vi "Laser Ethernet Rack_Init.vi"(0 "object in":refnum<class "Laser Ethernet Rack.lvclass">, 5 "error in (no error)":errorcluster) -> (14 "object out":refnum<class "Laser Ethernet Rack.lvclass">, 19 "error out":errorcluster)   [LabVIEW 2023, in "Laser Ethernet Rack.lvclass"]
uses:
  Laser Ethernet Rack.lvclass
  C:/Users/TimBerrier/Code/LabVIEW/Source/APIs/IPG/ipg_tcp/Laser_Ethernet_class/Laser_Ethernet.lvclass
  Laser Ethernet Rack.lvclass/Laser Ethernet Rack.ctl
  Laser_Ethernet_class/Laser_Ethernet.lvclass
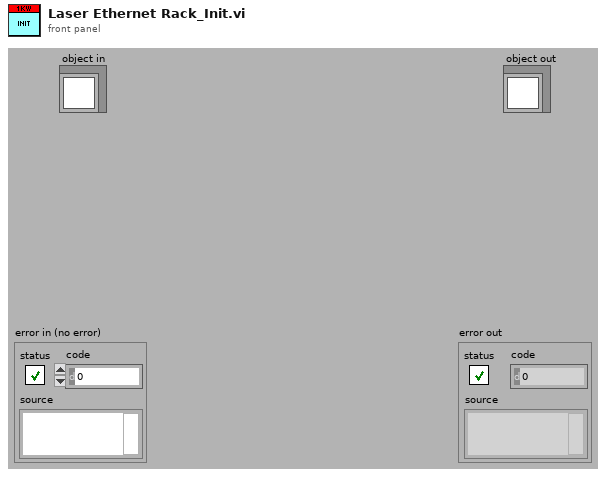
[diagram p1: front panel]
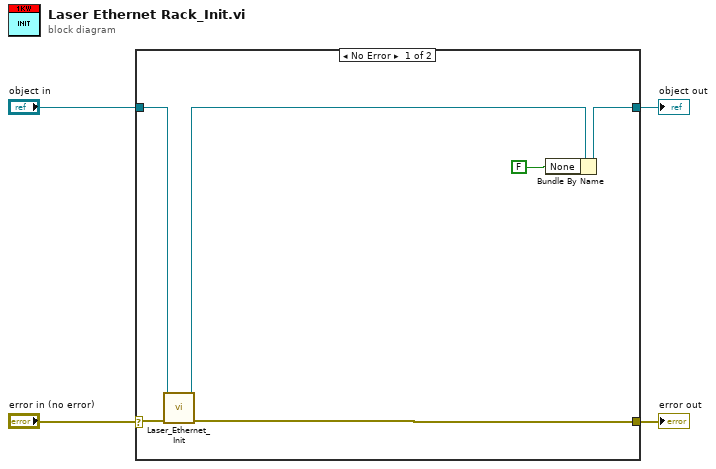
[diagram p0: block diagram]
diagram:
  n1 = case shown="No Error" "error in (no error)" {
    selector: "error in (no error)" -> [w8 w11]
    tunnel: [w10 w12] -> w4
    tunnel: "object in" -> [w6 w12]
    tunnel: [w7 w11] -> w1
    frame No Error {
      n2 = call "Laser_Ethernet_Init.vi"("error in (no error)"=w8, "object in"=w6) -> ("error out"=w7:errorcluster, "object out"=w5:refnum<class "Laser Ethernet Rack.lvclass">)  [unwired: 8 in]
      n3 = Bundle By Name(cluster=w5, "None"=FALSE) -> (w10:refnum<class "Laser Ethernet Rack.lvclass">)
    }
    frame Error {
    }
  }
  "object out" <- w4
  "error out" <- w1
